vi "ErrorQ.vi"(4 "command":T2, 5 "error in (no error)":errorcluster, 6 "DataIn":variant, 7 "ErrorMessage":T1) -> (0 "error out":errorcluster, 1 "DataOut":variant, 2 "ErrorMessageOut":T1, 3 "queue out":refnum<queue>)   [LabVIEW 2023]
doc: "*-----------------------------------------------------\n* Author: Swatts\n*\n* VI Description: Queue component for Error handling\n* \n*\n* Error handling: All errors passed out and sent to Q receiver\n*\n* Pre-condition: \n*\n* Post-condition: None\n*\n* Revision History:\n*\n* Rev Date Author Description \n* 01 29/04/2014 SWatts First issue\n*\n*-----------------------------------------------------"
uses:
  ErrorMessage.ctl
  Controls/DisplayQCommand.ctl
panel:
  # "Output"
  # "Input"
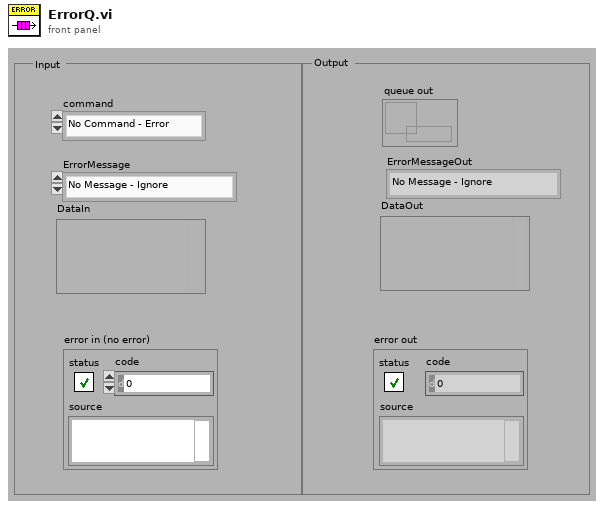
[diagram p1: front panel]
types:
  T1 = typedef "ErrorMessage.ctl" = enum16{"No Message - Ignore", "Display Message", "Stop"}
  T2 = typedef "DisplayQCommand.ctl" = enum16{"No Command - Error", "Initialise", "Get Q Reference", "Add Item to Bottom", "Add Item to Top", "Flush Q", "Dequeue", "Peek Next Element", "Close"}
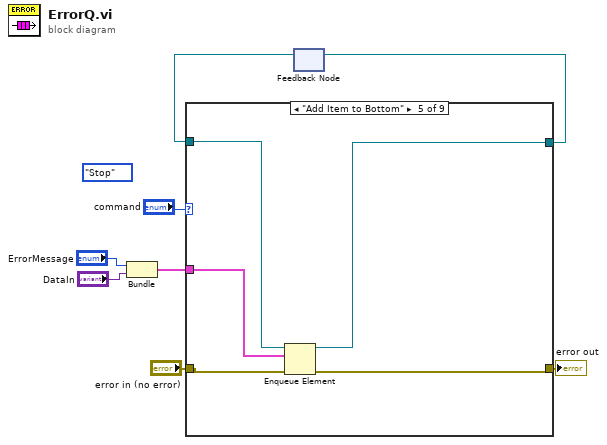
[diagram p0: block diagram]
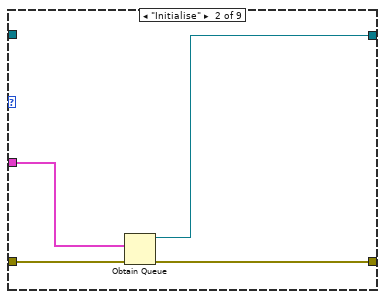
[diagram p3: hidden frame]
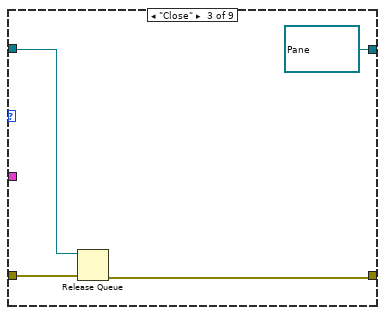
[diagram p4: hidden frame]
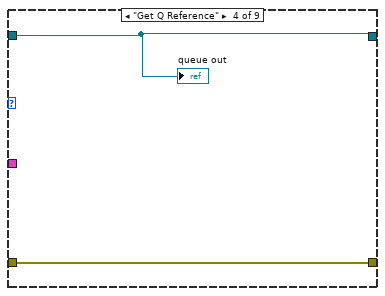
[diagram p5: hidden frame]
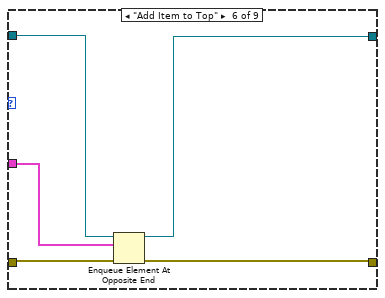
[diagram p6: hidden frame]
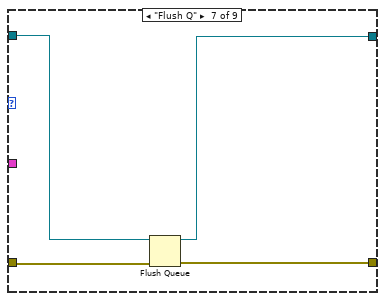
[diagram p7: hidden frame]
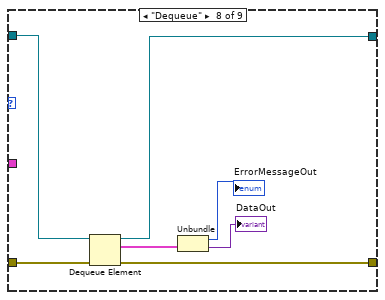
[diagram p8: hidden frame]
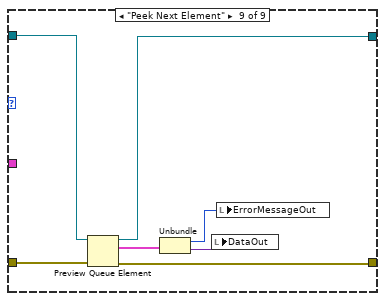
[diagram p9: hidden frame]
diagram:
  (unwired) ErrorMessage."Stop" ("ErrorMessage")
  n1 = Bundle("ErrorMessage"="ErrorMessage", "DataIn"="DataIn") -> (w1:cluster{"ErrorMessage":T1, "DataIn":variant})  [unwired: 1 in]
  n2 = feedback #1() -> (w4:refnum<queue>)  [unwired: 1 in]
  n3 = case shown="\"Add Item to Bottom\"" "command" {
    tunnel: "error in (no error)" -> [w9 w14 w18 w19 w25 w30 w31 w41 w48]
    tunnel: [w9 w13 w17 w19 w24 w29 w34 w39 w47] -> w6
    tunnel: [w10 w12 refnum<queue> refnum ("queue out") w20 w23 w27 w33 w38 w45] -> w5
    tunnel: w4 -> [w10 _ w16 w20 w22 w28 w32 w40 w46]
    tunnel: w1 -> [_ w11 _ _ w21 w26 _ _ _]
    frame "No Command - Error", Default {
    }
    frame "Initialise" {
      n4 = Obtain Queue(element data type=w11, error in (no error)=w14) -> (queue out=w12:refnum<queue>, error out=w13:errorcluster)  [unwired: 3 in, 1 out]
    }
    frame "Close" {
      n5 = Release Queue(queue=w16, error in (no error)=w18) -> (error out=w17:errorcluster)  [unwired: 1 in, 2 out]
    }
    frame "Get Q Reference" {
      "queue out" <- w20
    }
    frame "Add Item to Bottom" {
      n6 = Enqueue Element(queue=w22, element=w21, error in (no error)=w25) -> (queue out=w23:refnum<queue>, error out=w24:errorcluster)  [unwired: 1 in, 1 out]
    }
    frame "Add Item to Top" {
      n7 = Enqueue Element At Opposite End(queue=w28, element=w26, error in (no error)=w30) -> (queue out=w27:refnum<queue>, error out=w29:errorcluster)  [unwired: 1 in, 1 out]
    }
    frame "Flush Q" {
      n8 = Flush Queue(queue=w32, error in (no error)=w31) -> (queue out=w33:refnum<queue>, error out=w34:errorcluster)  [unwired: 1 out]
    }
    frame "Dequeue" {
      n9 = Dequeue Element(queue=w40, error in (no error)=w41) -> (queue out=w38:refnum<queue>, element=w37:cluster{"ErrorMessage":T1, "DataIn":variant}, error out=w39:errorcluster)  [unwired: 1 in, 1 out]
      n10 = Unbundle(w37) -> ("ErrorMessage"=→"ErrorMessageOut":T1, "DataIn"=→"DataOut":variant)
    }
    frame "Peek Next Element" {
      n11 = Preview Queue Element(queue=w46, error in (no error)=w48) -> (queue out=w45:refnum<queue>, element=w44:cluster{"ErrorMessage":T1, "DataIn":variant}, error out=w47:errorcluster)  [unwired: 1 in, 1 out]
      n12 = Unbundle(w44) -> ("ErrorMessage"=w43:T1, "DataIn"=w42:variant)
      n13 = local write "DataOut"(w42) -> ()
      n14 = local write "ErrorMessageOut"(w43) -> ()
    }
  }
  "error out" <- w6
  n15 = feedback-in #1(w5) -> ()
